vi "External Fan Command Test.vi"(8 "error in (no error)":errorcluster, 10 "Message IN":string) -> (0 "error out":errorcluster, 1 "Result (bool)":bool, 2 "Message OUT":string, 3 "VISA resource name 2":refnum<visa-resource-name>)   [LabVIEW 2022 SP3]
uses:
  <vilib>/DAQmx/write.llb/DAQmx Write (Digital Bool 1Line 1Point).vi
  <vilib>/DAQmx/read.llb/DAQmx Read (Digital Bool 1Line 1Point).vi
  <vilib>/DAQmx/miscellaneous.llb/DAQmx Fill In Error Info.vi
panel:
  out "DAQ Reading":bool
  out "Result (color)":u32(colorbox)
  out "LC DO Cmd":bool[](array[boolean])
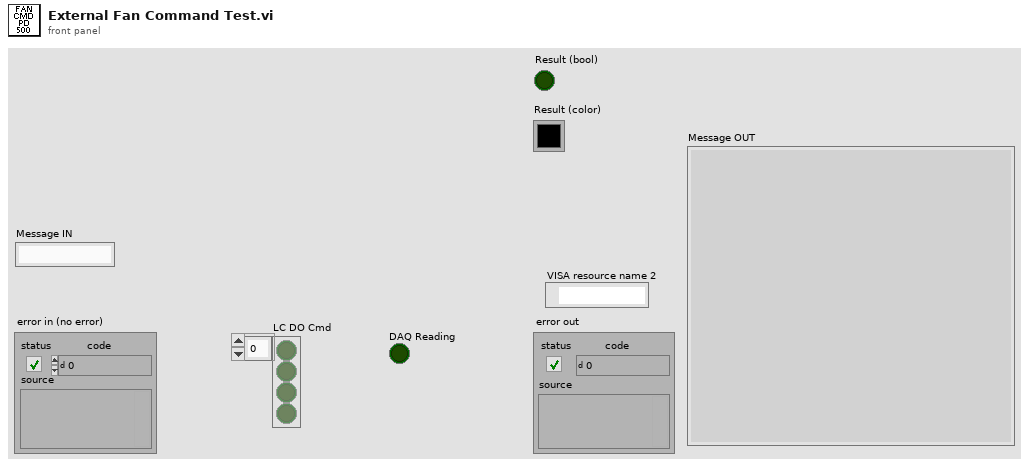
[diagram p1: front panel]
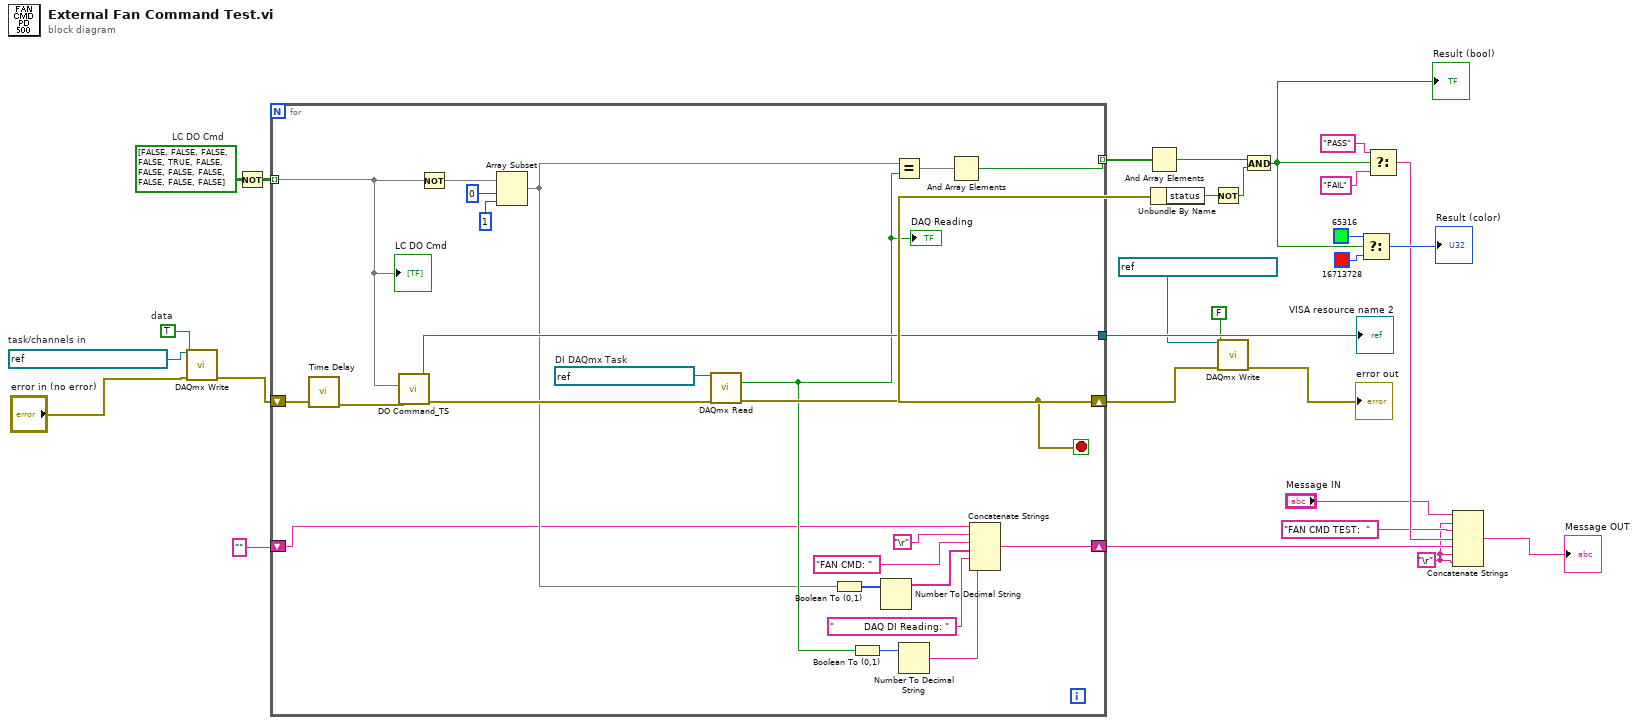
[diagram p0: block diagram]
diagram:
  w5 = TRUE  # data
  w6 = refnum<k21> "FTS2_ProgrammingRelay"  # task/channels in
  w10 = bool[][] [[FALSE, FALSE, FALSE, FALSE], [TRUE, FALSE, FALSE, FALSE], [FALSE, FALSE, FALSE, FALSE]]  # LC DO Cmd
  w12 = "\r"
  n1 = call-poly <vilib>:"DAQmx Write.vi"("task/channels in"=w6, "data"=w5, "error in"="error in (no error)") -> ("error out"=w7:errorcluster)  [unwired: 10 in, 2 out]
  n2 = Not(x=w10) -> (.not. x?=w9:bool[][])
  n3 = for {
    shift-right: [w47] -> w4
    shift-left: w7 -> [w30]
    tunnel: [w49] -> w27
    tunnel: [w51] -> w28 mode=indexing
    shift-right: [w38] -> w17
    shift-left: "" -> [w31]
    tunnel: w9 -> [w34] mode=indexing
    stop <- w47 stop-if-true
    w48 = refnum<k21> "FTS2_PD500_FanCmd"  # DI DAQmx Task
    n4 = call "Time Delay"("error in (no error)"=w30) -> ("error out"=w29:errorcluster)  [unwired: 10 in]
    n5 = call "DO Command_TS.vi"("error in (no error)"=w29, "DO Command"=w34) -> ("error out"=w37:errorcluster, "VISA Refnum out"=w49:refnum<visa-resource-name>)  [unwired: 8 in]
    n6 = Not(x=w34) -> (.not. x?=w32:bool[])
    n7 = Array Subset(array=w32, index=0, length=1) -> (w33:bool[])
    n8 = call-poly <vilib>:"DAQmx Read.vi"("task/channels in"=w48, "error in"=w37) -> ("data"=w39:bool, "error out"=w47:errorcluster)  [unwired: 11 in, 1 out]
    "DAQ Reading" <- w39
    n9 = Boolean To (0,1)(Boolean=w33) -> (0, 1=w41:i16[])
    n10 = Boolean To (0,1)(Boolean=w39) -> (0, 1=w40:i16)
    n11 = Number To Decimal String(number=w41) -> (decimal integer string=w44:string[])  [unwired: 1 in]
    n12 = Equal?(x=w33, y=w39) -> (x = y?=w50:bool[])
    n13 = Number To Decimal String(number=w40) -> (decimal integer string=w46:string)  [unwired: 1 in]
    n14 = And Array Elements(Boolean array=w50) -> (logical AND=w51:bool)
    n15 = Concatenate Strings(w31, "\r", "FAN CMD: ", w44, "          DAQ DI Reading: ", w46) -> (w38:string)
    "LC DO Cmd" <- w34
  }
  "VISA resource name 2" <- w27
  n16 = And Array Elements(Boolean array=w28) -> (logical AND=w18:bool)
  n17 = Unbundle By Name(w4) -> ("status"=w21:bool)
  n18 = Not(x=w21) -> (.not. x?=w20:bool)
  n19 = call-poly <vilib>:"DAQmx Write.vi"("task/channels in"=refnum<k21> "FTS2_ProgrammingRelay", "data"=FALSE, "error in"=w4) -> ("error out"=→"error out":errorcluster)  [unwired: 10 in, 2 out]
  n20 = And(x=w18, y=w20) -> (x .and. y?=w19:bool)
  "Result (bool)" <- w19
  n21 = Select(t=u32 65316 ("Result (color)"), s=w19, f=u32 16713728 ("Result (color)")) -> (s? t:f=→"Result (color)":u32)
  n22 = Select(t="PASS", s=w19, f="FAIL") -> (s? t:f=w15:string)
  n23 = Concatenate Strings("Message IN", w12, "FAN CMD TEST:  ", w15, w17, w12, w12) -> (→"Message OUT":string)
